vi "OperationOne.vi"(8 "error in (no error)":errorcluster, 11 "ProductB":refnum<class "ProductB.lvclass">) -> (0 "error out":errorcluster, 2 "ResultString":string, 3 "ProductB":refnum<class "ProductB.lvclass">)   [LabVIEW 2020, in "FactoryMethod.lvlib" / "FactoryMethodLazyEvaluation.lvlib" / "ProductB.lvclass"]
uses:
  ProductB.lvclass
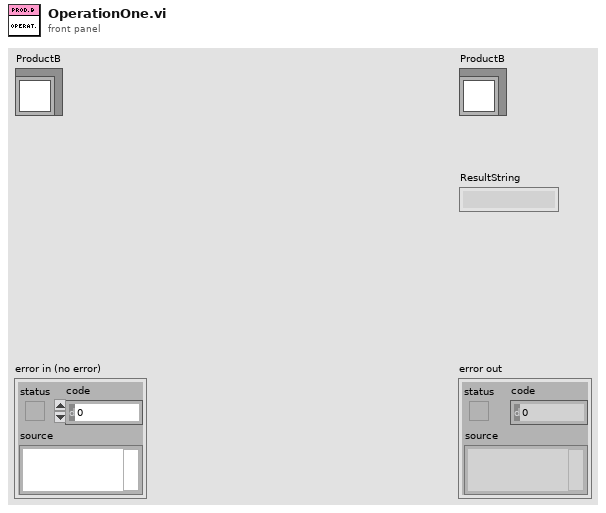
[diagram p1: front panel]
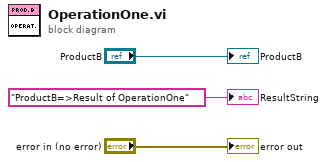
[diagram p0: block diagram]
diagram:
  "error out" <- "error in (no error)"
  "ProductB" <- "ProductB"
  "ResultString" <- "ProductB=>Result of OperationOne" ("ResultString")
